vi "niScope Read (poly).vi"   [LabVIEW 2011]
doc: "Inititates an acquisition, waits for it to complete, and acquires data."
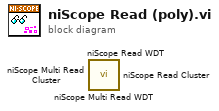
[diagram p0: block diagram]
diagram:
  n1 = call <instrlib>:"niScope Multi Read WDT.vi"() -> ()  [unwired: 8 in, 4 out]
  n2 = call <instrlib>:"niScope Read WDT.vi"() -> ()  [unwired: 8 in, 4 out]
  n3 = call <instrlib>:"niScope Multi Read Cluster.vi"() -> ()  [unwired: 8 in, 4 out]
  n4 = call <instrlib>:"niScope Read Cluster.vi"() -> ()  [unwired: 8 in, 4 out]
